vi "Detect Framework From Application Domain.vi"(8 "error in (no error)":errorcluster) -> (0 "error out":errorcluster, 1 "Test Framework Instance":refnum<class "Test Framework.lvclass">, 2 "Test Framework Type":T1=enum."LVUnit")   [LabVIEW 2017, in "Transparent Assertions.lvlib" / "Frameworks.lvlib" / "Test Framework Factory.lvclass"]
uses:
  Test Framework Factory.lvclass
  Test Framework/Test Framework.lvclass
  Test Framework.ctl
  Frameworks.lvlib
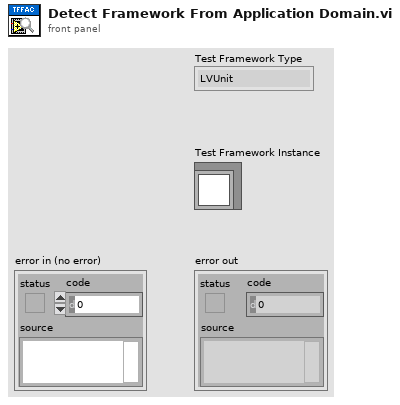
[diagram p1: front panel]
types:
  T1 = typedef "Transparent Assertions.lvlib/Frameworks.lvlib/Test Framework.ctl" = enum16{"Unknown", "LVUnit", "Caraya"}
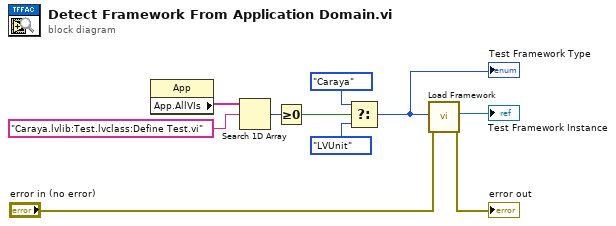
[diagram p0: block diagram]
diagram:
  n1 = property class="App"() -> ("App.AllVIs"=w10:string[])  [unwired: 2 in, 2 out]
  n2 = Search 1D Array(1D array=w10, element="Caraya.lvlib:Test.lvclass:Define Test.vi") -> (index of element=w8:i32)  [unwired: 1 in]
  n3 = Greater Or Equal To 0?(x=w8) -> (x >= 0?=w7:bool)
  n4 = Select(t=Test_Framework."Caraya" ("Test Framework Type"), s=w7, f=Test_Framework."LVUnit" ("Test Framework Type")) -> (s? t:f=w3:T1)
  "Test Framework Type" <- w3
  n5 = call "Load Framework.vi"("error in (no error)"="error in (no error)", "Test Framework Type"=w3) -> ("error out"=→"error out":errorcluster, "Test Framework Instance"=→"Test Framework Instance":refnum<class "Test Framework.lvclass">)  [unwired: 8 in]
